vi "XY Graph Get Plot Number.vi"(2 "XYGraph":refnum<vi>) -> (7 "# Plots":i32)   [LabVIEW 2019]
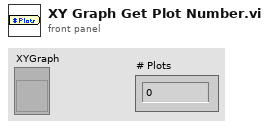
[diagram p1: front panel]
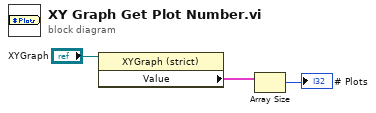
[diagram p0: block diagram]
diagram:
  n1 = property class="XYGraph (strict)"(reference="XYGraph") -> ("Value"=w2:cluster{"X Array":dbl[], "Y Array":dbl[]}[])  [unwired: 1 in, 2 out]
  n2 = Array Size(array=w2) -> (size(s)=→"# Plots":i32)
